vi "标签提交.vi"(8 "error in":errorcluster caption="错误输入（无错误）", 9 "附注":string, 10 "标签（版本）":string, 11 "仓库路径":path=path "E:/学习文件/Git插件/test") -> (0 "error out":errorcluster caption="错误输出", 1 "standard error":string caption="标准错误", 2 "standard output":string caption="标准输出", 3 "仓库路径":path=path "E:/学习文件/Git插件/test")   [LabVIEW 2018]
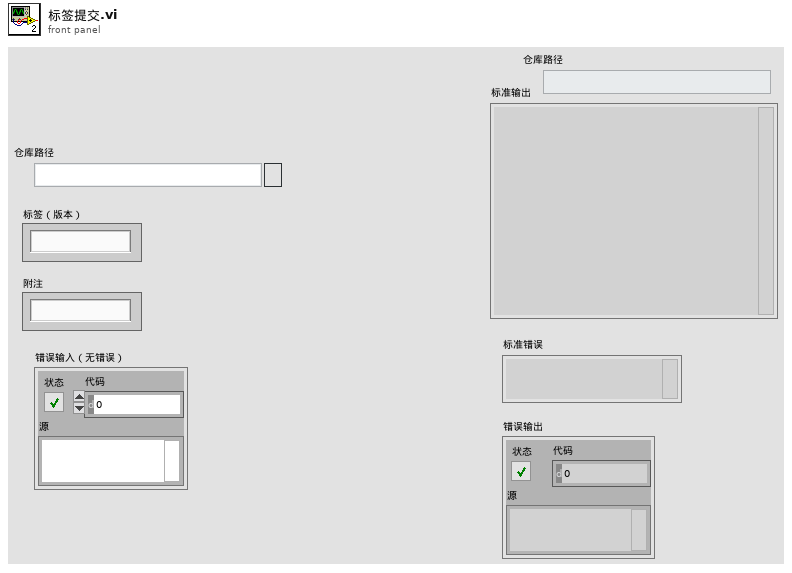
[diagram p1: front panel]
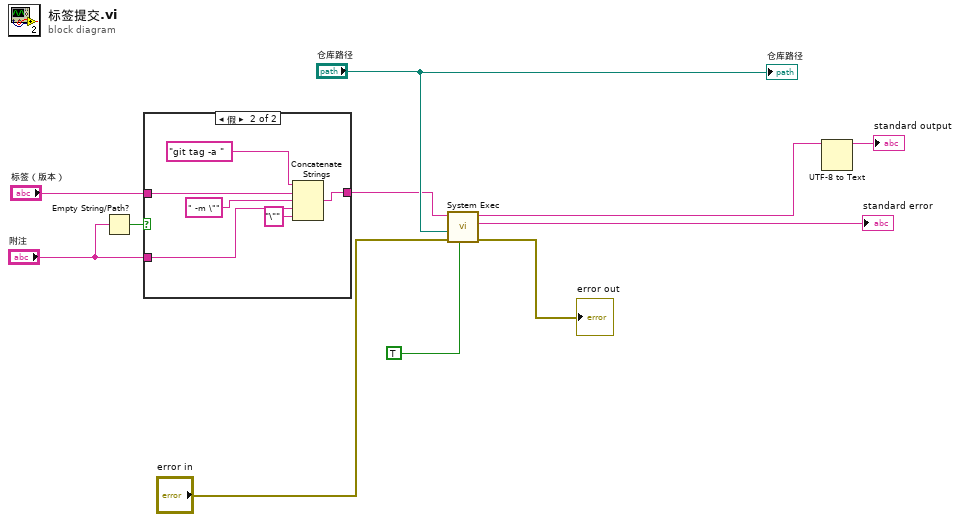
[diagram p0: block diagram]
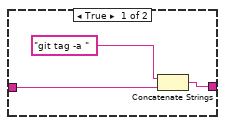
[diagram p2: hidden frame]
diagram:
  n1 = Empty String/Path?(string/path="附注") -> (empty?=w2:bool)
  n2 = case shown="假" w2 {
    tunnel: "标签（版本）" -> [w13 w18]
    tunnel: [w12 w17] -> w3
    tunnel: "附注" -> [_ w16]
    frame True {
      n3 = Concatenate Strings("git tag -a " ("command line"), w13) -> (w12:string)
    }
    frame False {
      n4 = Concatenate Strings("git tag -a " ("command line"), w18, " -m \"" ("字符串"), w16, "\"" ("字符串")) -> (w17:string)
    }
  }
  n5 = call <vilib>:"System Exec.vi"("run minimized? (F)"=TRUE, "error in (no error)"="error in", "working directory"="仓库路径", "command line"=w3) -> ("error out"=→"error out":errorcluster, "standard error"=→"standard error":string, "standard output"=w10:string)  [unwired: 4 in, 1 out]
  n6 = UTF-8 to Text ("UTF-8至文本转换")(11:w10) -> (3:→"standard output":string)  [unwired: 2 in, 1 out]
  "仓库路径" <- "仓库路径"
